vi "PartChangeLine(SubVI).vi"(7 "element in":T1 {"Color" format="%x"}, 8 "error in (no error)":errorcluster, 9 "Arr Refnum":refnum<vi>, 10 "String in":string, 11 "ComboBox in":refnum<vi>) -> (0 "error out":errorcluster, 2 "NumPlot":dbl, 3 "element out":T1 {"Color" format="%x"})   [LabVIEW 2018]
uses:
  CTL/Line.ctl
  Windows/Settings/View.ctl
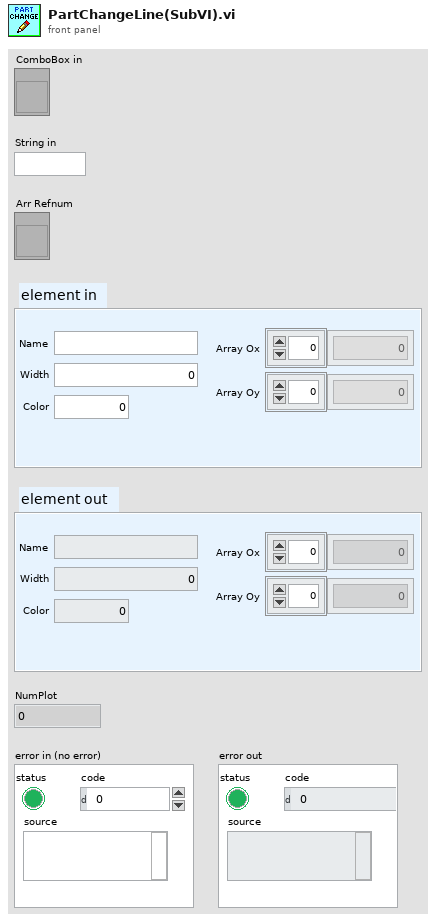
[diagram p1: front panel]
types:
  T1 = typedef "Line.ctl" = cluster{"Width":dbl, "Color":i64, "Array Oy":dbl[], "Array Ox":dbl[], "Name":string, "Plot Visible":T2}
  T2 = typedef "View.ctl" = bool
  T3 = typedef "LVComboBoxStrsAndValuesArrayTypeDef.ctl" = cluster{"String":string, "Value":string}[]
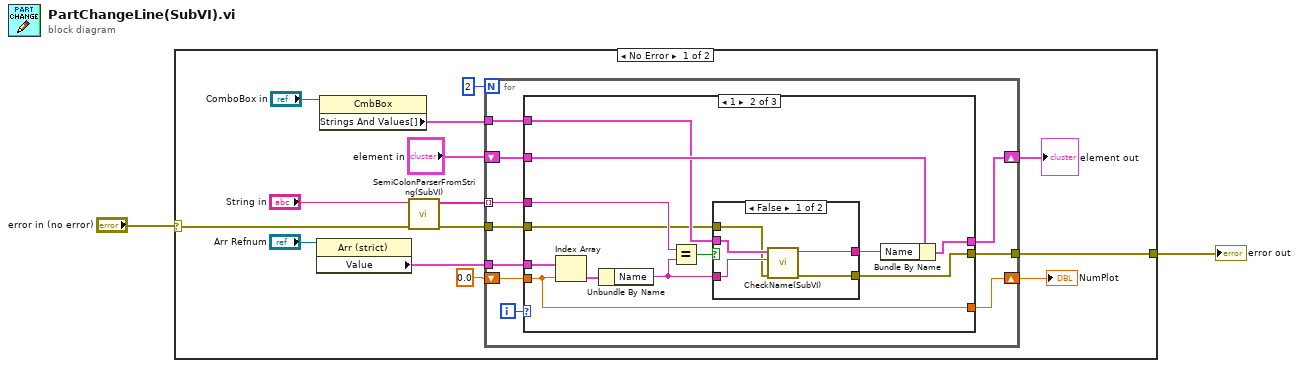
[diagram p0: block diagram]
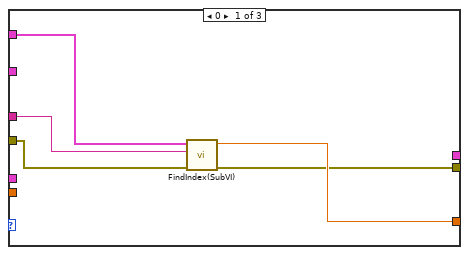
[diagram p2: hidden frame]
diagram:
  n1 = case shown="No Error" "error in (no error)" {
    selector: "error in (no error)" -> [w6 w52]
    tunnel: [w4 w52] -> w1
    frame No Error {
      n2 = property on="Property Node" class="Arr (strict)"(reference="Arr Refnum") -> ("Value"=w8:T1[])  [unwired: 1 in, 2 out]
      n3 = property on="Property Node" class="CmbBox"(reference="ComboBox in") -> ("Strings And Values[]"=w9:T3)  [unwired: 1 in, 2 out]
      n4 = call "SemiColonParserFromString(SubVI).vi"("Error In"=w6, "String In"="String in") -> ("Error Out"=w5:errorcluster, "String Array Out"=w7:string[])  [unwired: 8 in]
      n5 = for {
        N: 2 -> [_]
        shift-right: [w25] -> w14
        shift-left: "element in" -> [w24]
        shift-right: [w23] -> w16
        shift-left: 0.0 ("NumPlot") -> [w21]
        tunnel: w8 -> [w22]
        tunnel: w9 -> [w20]
        tunnel: w7 -> [w19] mode=indexing
        tunnel: w5 -> [w18]
        tunnel: [w17] -> w4
        i -> [w26]
        n6 = case shown="1" w26 {
          tunnel: [_ w38 _] -> w25
          tunnel: w24 -> [_ w39 _]
          tunnel: [w31 w37 _] -> w23
          tunnel: w22 -> [_ w41 _]
          tunnel: w21 -> [_ w37 _]
          tunnel: w20 -> [w30 w36 _]
          tunnel: w19 -> [w29 w35 _]
          tunnel: w18 -> [w28 w33 w51]
          tunnel: [w27 w32 w51] -> w17
          frame 0 {
            n7 = call "FindIndex(SubVI).vi"("Error In"=w28, "Name"=w29, "Strings And Values[]"=w30) -> ("Error Out"=w27:errorcluster, "Index"=w31:dbl)  [unwired: 7 in]
          }
          frame 1 {
            n8 = Index Array(array=w41, index=w37) -> (element=w43:T1)
            n9 = Unbundle By Name(w43) -> ("Name"=w34:string)
            n10 = Equal?(x=w35, y=w34) -> (x = y?=w42:bool)
            n11 = case shown="False" w42 {
              tunnel: w36 -> [w48 _]
              tunnel: [w47 w50] -> w40
              tunnel: w34 -> [w46 w50]
              tunnel: w33 -> [w45 w49]
              tunnel: [w44 w49] -> w32
              frame False {
                n12 = call "CheckName(SubVI).vi"("Error In"=w45, "Name In"=w46, "Strings And Values[]"=w48) -> ("Error Out"=w44:errorcluster, "Name Out"=w47:string)  [unwired: 7 in]
              }
              frame True {
              }
            }
            n13 = Bundle By Name(cluster=w39, "Name"=w40) -> (w38:T1)
          }
          frame Default {
          }
        }
      }
      "NumPlot" <- w16
      "element out" <- w14
    }
    frame Error {
    }
  }
  "error out" <- w1
